vi "Organise_measurements.vi"(0 "VISA resource name":refnum<visa-resource-name>, 1 "Sweep 0":T1={"DorG_0"="", "Vvar_0_start"=0.0, "Vvar_0_step"=0.0, "Vvar_0_Stop"=0.0, "Vvar_1_start "=0.0, "Drain Current Compliance"=1e-06, "Gate Current Compliance 0"=1e-06, "Vvar_0_holdtime"=0.0, "Vvar-0_delaytime"=0.0, "IntPts_0"=100.0, "Set Swe_0_Mode"="", "Sweep Spacing_0"=""}, 2 "Sweep 1_replac":T1={"DorG_0"="", "Vvar_0_start"=0.0, "Vvar_0_step"=0.0, "Vvar_0_Stop"=0.0, "Vvar_1_start "=0.0, "Drain Current Compliance"=1e-06, "Gate Current Compliance 0"=1e-06, "Vvar_0_holdtime"=0.0, "Vvar-0_delaytime"=0.0, "IntPts_0"=100.0, "Set Swe_0_Mode"="", "Sweep Spacing_0"=""}, 3 "Sweep 2_replac 2":T1={"DorG_0"="", "Vvar_0_start"=0.0, "Vvar_0_step"=0.0, "Vvar_0_Stop"=0.0, "Vvar_1_start "=0.0, "Drain Current Compliance"=1e-06, "Gate Current Compliance 0"=1e-06, "Vvar_0_holdtime"=0.0, "Vvar-0_delaytime"=0.0, "IntPts_0"=100.0, "Set Swe_0_Mode"="", "Sweep Spacing_0"=""}, 5 "Sweep 0":bool, 7 "Sweep 2":bool, 9 "# Cycles":dbl, 11 "error in (no error)":errorcluster, 12 "SMU1 Terminal":string(combo)="Source") -> (4 "VISA resource name out":refnum<visa-resource-name>, 8 "WarmUp":dbl[][](array[numeric]), 10 "Recorded_Data":dbl[][][](array[numeric]), 15 "error out":errorcluster)   [LabVIEW 2021]
panel:
  # "Output from organise Measurement"
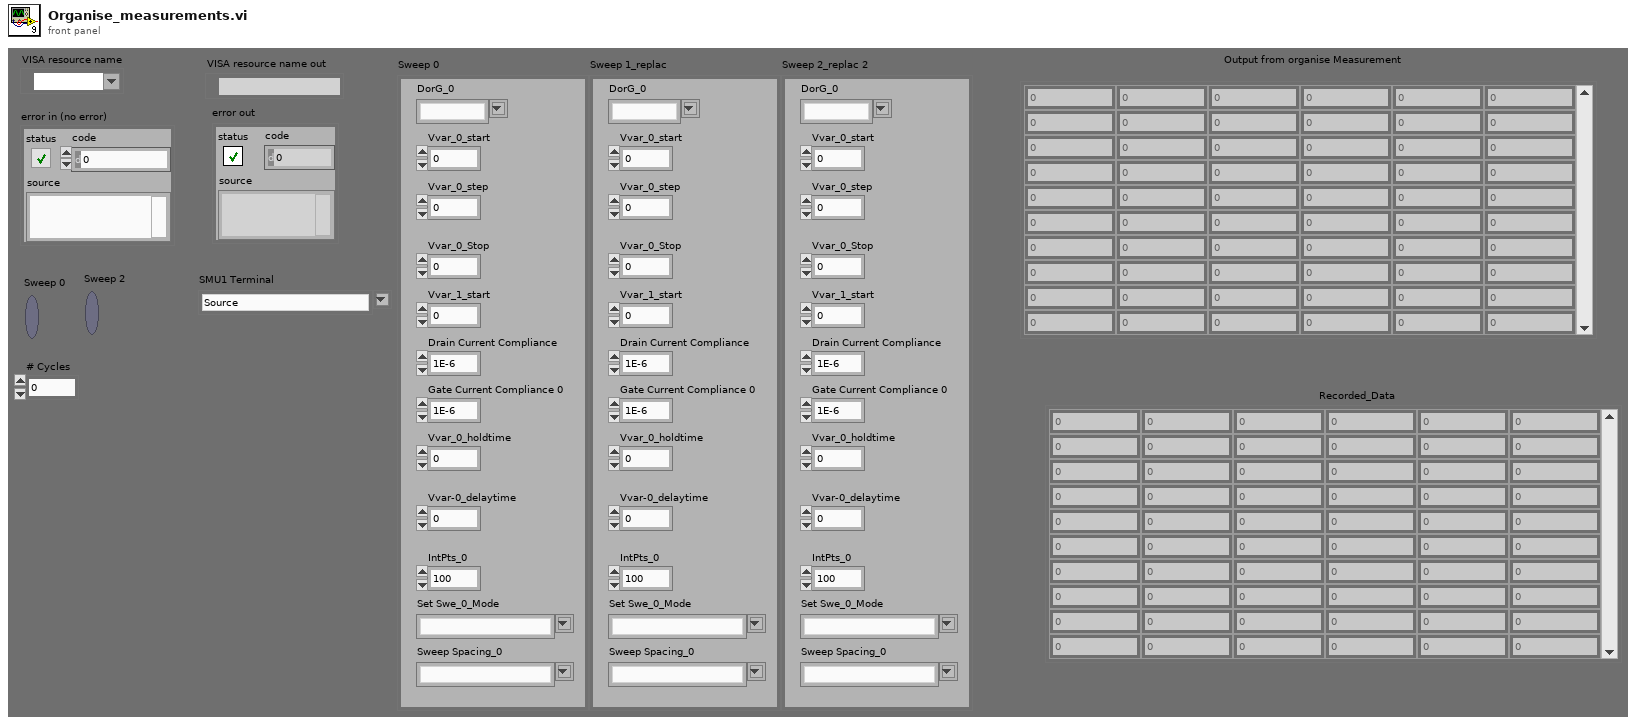
[diagram p1: front panel]
types:
  T1 = cluster{"DorG_0":string, "Vvar_0_start":dbl, "Vvar_0_step":dbl, "Vvar_0_Stop":dbl, "Vvar_1_start ":dbl, "Drain Current Compliance":dbl, "Gate Current Compliance 0":dbl, "Vvar_0_holdtime":dbl, "Vvar-0_delaytime":dbl, "IntPts_0":dbl, "Set Swe_0_Mode":string, "Sweep Spacing_0":string}
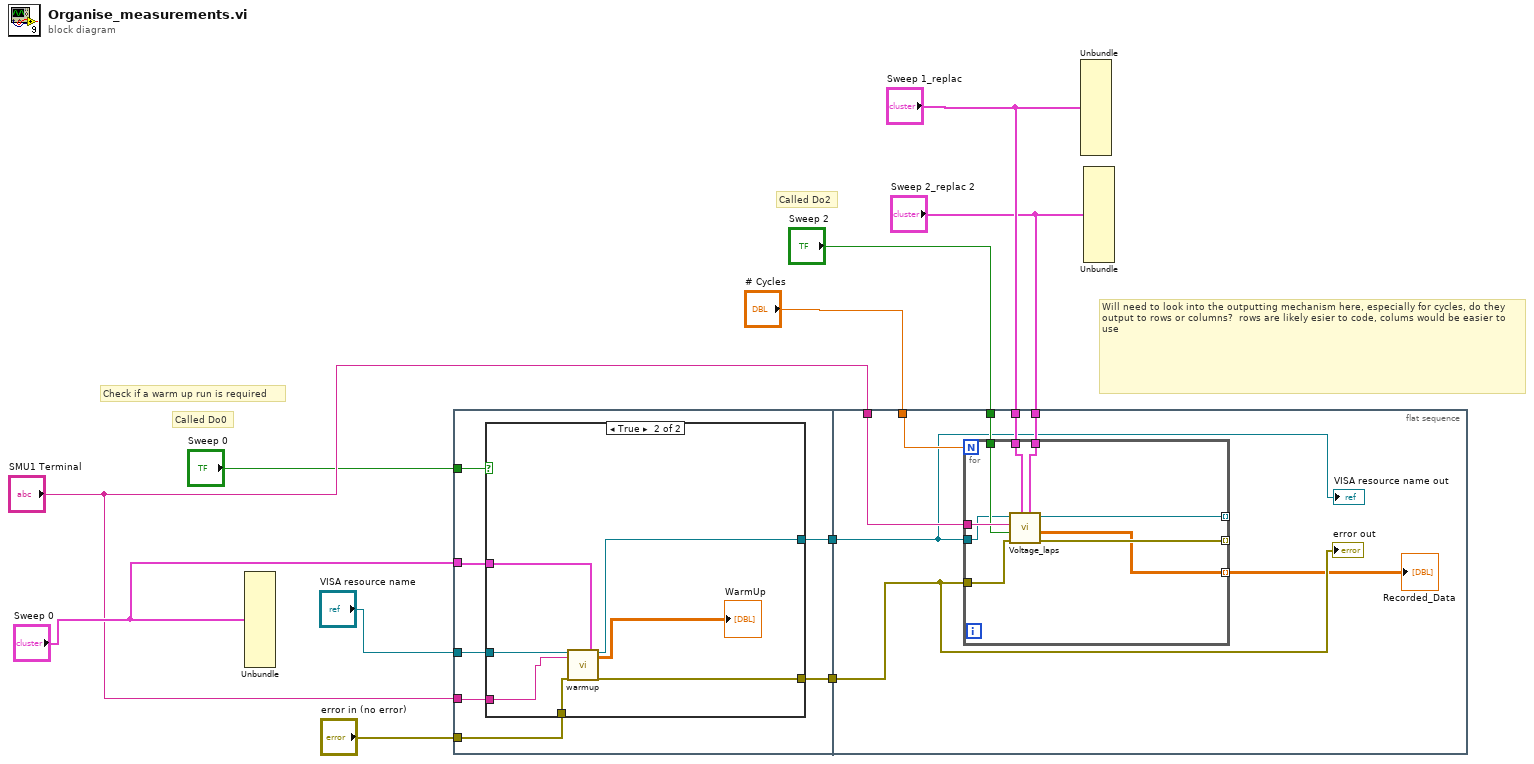
[diagram p0: block diagram]
diagram:
  # "Will need to look into the outputting mechanism here, especially for cycles, do they output to rows or columns?  rows are likely esier to code, colums would be easier to use"
  # "Check if a warm up run is required"
  # "Called Do2"
  # "Called Do0"
  n1 = Unbundle("Sweep 0") -> ()  [unwired: 12 out]
  n2 = flat-sequence {
    tunnel: "Sweep 0" -> [w18]
    tunnel: "SMU1 Terminal" -> [w17]
    tunnel: "Sweep 0" -> [w16]
    tunnel: [w15] -> w6
    tunnel: [w14] -> w5
    tunnel: "VISA resource name" -> [w13]
    tunnel: "error in (no error)" -> [w12]
    tunnel: "# Cycles" -> [w35]
    tunnel: "Sweep 1_replac" -> [w34]
    tunnel: "Sweep 2_replac 2" -> [w33]
    tunnel: "SMU1 Terminal" -> [w32]
    tunnel: "Sweep 2" -> [w31]
    tunnel: w6 -> [w29]
    tunnel: w5 -> [w30]
    frame #0 {
      n3 = case shown="True" w16 {
        tunnel: w18 -> [_ w27]
        tunnel: w17 -> [_ w26]
        tunnel: [w20 w24] -> w15
        tunnel: [w19 w23] -> w14
        tunnel: w13 -> [w20 w22]
        tunnel: w12 -> [w19 w21]
        frame False {
        }
        frame True {
          n4 = call "warmup.vi"("VISA resource name"=w22, "SMU1 Terminal"=w26, "error in (no error)"=w21, "Sweep 0"=w27) -> ("VISA resource name out"=w24:refnum<visa-resource-name>, "Recorded_data"=→"WarmUp":dbl[][], "error out"=w23:errorcluster)  [unwired: 13 in]
        }
      }
    }
    frame #1 {
      n5 = for {
        N: w35 -> [_]
        tunnel: w34 -> [w44]
        tunnel: w33 -> [w43]
        tunnel: w32 -> [w42]
        tunnel: w31 -> [w41]
        tunnel: w29 -> [w40]
        tunnel: w30 -> [w39]
        tunnel: [w38] -> _ mode=indexing
        tunnel: [w37] -> _ mode=indexing
        tunnel: [w36] -> w28 mode=indexing
        n6 = call "Voltage_laps.vi"(4:"Sweep 2"=w43, "Sweep 1"=w44, "error in (no error)"=w39, 7:"Sweep 2"=w41, "smu_1_port"=w42, "VISA resource name"=w40) -> ("error out"=w37:errorcluster, "Recorded_data"=w36:dbl[][], "VISA resource name out"=w38:refnum<visa-resource-name>)  [unwired: 1 in]
      }
      "Recorded_Data" <- w28
      "VISA resource name out" <- w29
      "error out" <- w30
    }
  }
  n7 = Unbundle("Sweep 1_replac") -> ()  [unwired: 12 out]
  n8 = Unbundle("Sweep 2_replac 2") -> ()  [unwired: 12 out]
